vi "PRO LP Filter.vi"(7 "Fitler TC":dbl, 10 "In N -1":dbl, 11 "In N":dbl) -> (0 "Rindex":i16, 1 "XSwitch":bool, 2 "In Range?":bool, 3 "Filtered Out":dbl)   [LabVIEW 2024]
panel:
  out "Boolean":bool
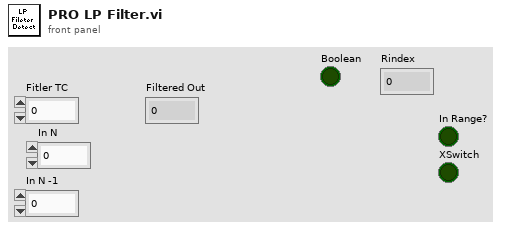
[diagram p1: front panel]
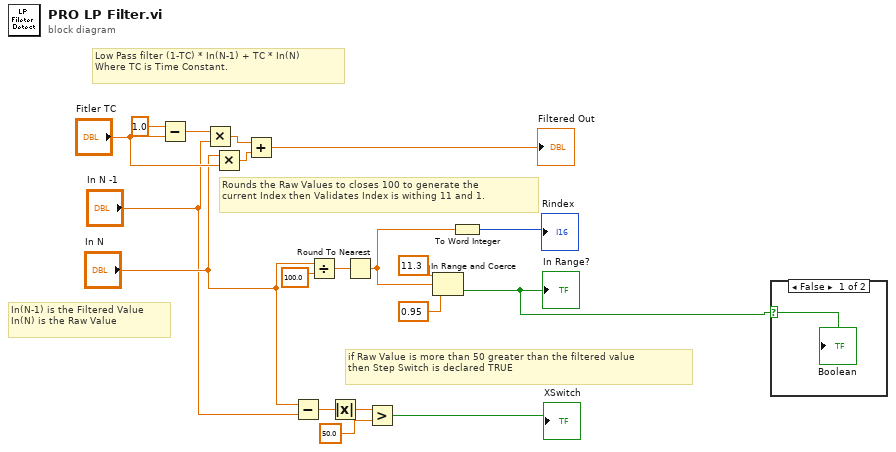
[diagram p0: block diagram]
diagram:
  # "if Raw Value is more than 50 greater than the filtered value\nthen Step Switch is declared TRUE"
  # "Rounds the Raw Values to closes 100 to generate the \ncurrent Index then Validates Index is withing 11 and 1."
  # "In(N-1) is the Filtered Value\nIn(N) is the Raw Value"
  # "Low Pass filter (1-TC) * In(N-1) + TC * In(N)\nWhere TC is Time Constant."
  n1 = Subtract(x=1.0, y="Fitler TC") -> (x-y=w14:dbl)
  n2 = Multiply(x=w14, y="In N -1") -> (x*y=w17:dbl)
  n3 = Multiply(x="In N", y="Fitler TC") -> (x*y=w16:dbl)
  n4 = Add(x=w17, y=w16) -> (x+y=→"Filtered Out":dbl)
  n5 = Subtract(x="In N", y="In N -1") -> (x-y=w13:dbl)
  n6 = Divide(x="In N", y=100.0) -> (x/y=w10:dbl)
  n7 = Absolute Value(x=w13) -> (abs(x)=w12:dbl)
  n8 = Round To Nearest(number=w10) -> (nearest integer value=w3:dbl)
  n9 = Greater?(x=w12, y=50.0) -> (0:→"XSwitch":bool)
  n10 = In Range and Coerce(upper limit=11.3, x=w3, lower limit=0.95) -> (In Range?=w1:bool)  [unwired: 1 out]
  "In Range?" <- w1
  n11 = To Word Integer(number=w3) -> (16bit integer=→"Rindex":i16)
  n12 = case shown="False" w1 {
    selector: w1 -> [w20 _]
    frame False {
      "Boolean" <- w20
    }
    frame True {
    }
  }
